vi "test_Gen_Square.vi"() -> ()   [LabVIEW 2023]
uses:
  projets/Capteur virtuel/VGS.ctl
panel:
  in  "VGS 2":T1={"Rapport cyclique (%)"=50.0, "Fréquence (Hz)"=50.0, "Phase (°)"=50.0, "V_H (V)"=50.0, "VL_(V)"=50.0} {"VL_(V)" format="%0.2f"; "V_H (V)" format="%0.2f"; "Phase (°)" format="%0.2f"; "Fréquence (Hz)" format="%0.2f"; "Rapport cyclique (%)" format="%0.2f"}
  in  "Tparam":cluster{"Freq ech (Hz)":dbl, "Temps (s)":dbl}={"Freq ech (Hz)"=50.0, "Temps (s)"=50.0} {"Temps (s)" format="%0.2f"; "Freq ech (Hz)" format="%0.2f"}
  out "Waveform Graph":dbl[][](graph)
  in  "VGS":T1={"Rapport cyclique (%)"=50.0, "Fréquence (Hz)"=50.0, "Phase (°)"=50.0, "V_H (V)"=50.0, "VL_(V)"=50.0} {"VL_(V)" format="%0.2f"; "V_H (V)" format="%0.2f"; "Phase (°)" format="%0.2f"; "Fréquence (Hz)" format="%0.2f"; "Rapport cyclique (%)" format="%0.2f"}
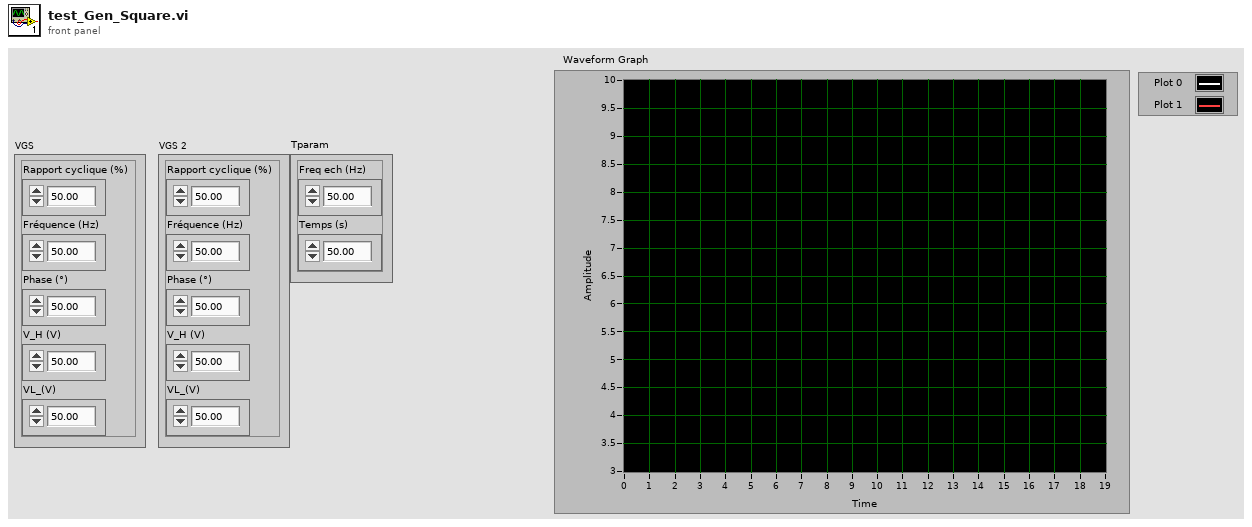
[diagram p1: front panel]
types:
  T1 = typedef "VGS.ctl" = cluster{"Rapport cyclique (%)":dbl, "Fréquence (Hz)":dbl, "Phase (°)":dbl, "V_H (V)":dbl, "VL_(V)":dbl}
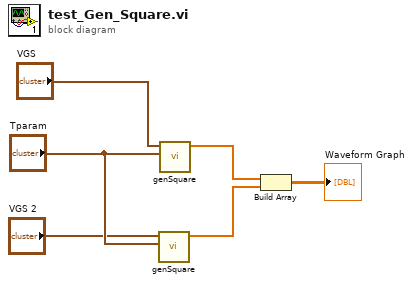
[diagram p0: block diagram]
diagram:
  n1 = call "genSquare.vi"("Tparam"="Tparam", "VGS"="VGS 2") -> ("Signal OUT"=w1:dbl[])  [unwired: 9 in]
  n2 = call "genSquare.vi"("Tparam"="Tparam", "VGS"="VGS") -> ("Signal OUT"=w6:dbl[])  [unwired: 9 in]
  n3 = Build Array(w6, w1) -> (→"Waveform Graph":dbl[][])
